vi "LassoLarsCV.vi"(8 "error in":errorcluster) -> (0 "error out":errorcluster, 3 "out":refnum<class "LassoLarsCV.lvclass">)   [LabVIEW 2020]
doc: "Cross-validated Lasso, using the LARS algorithm.\n\n See glossary entry for :term:`cross-validation estimator`.\n\n The optimization objective for Lasso is::\n\n (1 / (2 * n_samples)) * ||y - Xw||^2_2 + alpha * ||w||_1\n\n Read more in the :ref:`User Guide <least_angle_regression>`.\n\n Parameters\n ----------\n fit_intercept : bool, default=True\n whether to calculate the intercept for this model. If set\n to false, no intercept will be used in calculations\n (i.e. data is expected to be centered).\n\n verbose : bool or int, default=False\n Sets the verbosity amount.\n\n max_iter : int, default=500\n Maximum number of iterations to perform.\n\n normalize : bool, default=True\n This parameter is ignored when ``fit_intercept`` is set to False.\n If True, the regressors X will be normalized before regression by\n subtracting the mean and dividing by the l2-norm.\n If you wish to standardize, please use\n :class:`~sklearn.preprocessing.StandardScaler` before calling ``fit``\n on an estimator with ``normalize=False``.\n\n precompute : bool or 'auto' , default='auto'\n Whether to use a precomputed Gram matrix to speed up\n calculations. If set to ``'auto'`` let us decide. The Gram matrix\n cannot be passed as argument since we will use only subsets of X.\n\n cv : int, cross-validation generator or an iterable, default=None\n Determines the cross-validation splitting strategy.\n Possible inputs for cv are:\n\n - None, to use the default 5-fold cross-validation,\n - integer, to specify the number of folds.\n - :term:`CV splitter`,\n - An iterable yielding (train, test) splits as arrays of indices.\n\n For integer/None inputs, :class:`KFold` is used.\n\n Refer :ref:`User Guide <cross_validation>` for the various\n cross-validation strategies that can be used here.\n\n .. versionchanged:: 0.22\n ``cv`` default value if None changed from 3-fold to 5-fold.\n\n max_n_alphas : int, default=1000\n The maximum number of points on the path used to compute the\n residuals in the cross-validation\n\n n_jobs : int or None, default=None\n Number of CPUs to use during the cross validation.\n ``None`` means 1 unless in a :obj:`joblib.parallel_backend` context.\n ``-1`` means using all processors. See :term:`Glossary <n_jobs>`\n for more details.\n\n eps : float, default=np.finfo(float).eps\n The machine-precision regularization in the computation of the\n Cholesky diagonal factors. Increase this for very ill-conditioned\n systems. Unlike the ``tol`` parameter in some iterative\n optimization-based algorithms, this parameter does not control\n the tolerance of the optimization.\n\n copy_X : bool, default=True\n If True, X will be copied; else, it may be overwritten.\n\n positive : bool, default=False\n Restrict coefficients to be >= 0. Be aware that you might want to\n remove fit_intercept which is set True by default.\n Under the positive restriction the model coefficients do not converge\n to the ordinary-least-squares solution for small values of alpha.\n Only coefficients up to the smallest alpha value (``alphas_[alphas_ >\n 0.].min()`` when fit_path=True) reached by the stepwise Lars-Lasso\n algorithm are typically in congruence with the solution of the\n coordinate descent Lasso estimator.\n As a consequence using LassoLarsCV only makes sense for problems where\n a sparse solution is expected and/or reached.\n\n Attributes\n ----------\n coef_ : array-like of shape (n_features,)\n parameter vector (w in the formulation formula)\n\n intercept_ : float\n independent term in decision function.\n\n coef_path_ : array-like of shape (n_features, n_alphas)\n the varying values of the coefficients along the path\n\n alpha_ : float\n the estimated regularization parameter alpha\n\n alphas_ : array-like of shape (n_alphas,)\n the different values of alpha along the path\n\n cv_alphas_ : array-like of shape (n_cv_alphas,)\n all the values of alpha along the path for the different folds\n\n mse_path_ : array-like of shape (n_folds, n_cv_alphas)\n the mean square error on left-out for each fold along the path\n (alpha values given by ``cv_alphas``)\n\n n_iter_ : array-like or int\n the number of iterations run by Lars with the optimal alpha.\n\n active_ : list of int\n Indices of active variables at the end of the path.\n\n \nAvailable methods:\nGet Attributes\nGet Params\nSet Params"
uses:
  LassoLarsCV.lvclass
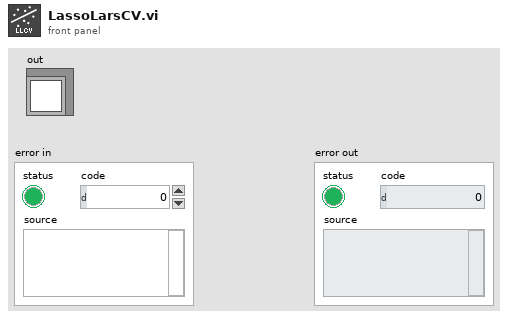
[diagram p1: front panel]
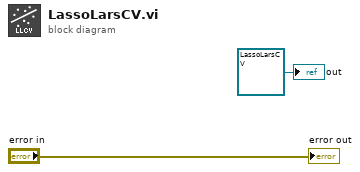
[diagram p0: block diagram]
diagram:
  "out" <- refnum<class "LassoLarsCV.lvclass"> refnum ("model")
  "error out" <- "error in"
